vi "Write to File.vi"(8 "error in (no error)":errorcluster, 10 "INI Ref":T1, 11 "Window Action in":refnum<class "Window Action.lvclass">) -> (0 "error out":errorcluster, 2 "INI Ref out":T1, 3 "Window Action out":refnum<class "Window Action.lvclass">)   [LabVIEW 2020, in "MacroAssert.lvlib" / "Window Action.lvclass"]
doc: "Writes associated parameters to the file identified by <B>INI Ref</B>."
uses:
  Window Action.lvclass
  C:/Users/User/Documents/LabVIEW Data/Projects/MacroAssert/source/Classes/Step/Step.lvclass
  <vilib>/Utility/config.llb/Config Data RefNum.ctl
  <vilib>/Utility/error.llb/Error Cluster From Error Code.vi
  <vilib>/Utility/config.llb/Write Key (String).vi
  Action Step/Action Step.lvclass
  MacroAssert.lvlib
  <vilib>/Utility/config.llb/NI_LVConfig.lvlib
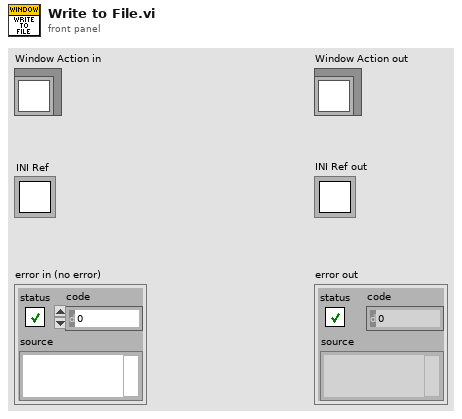
[diagram p1: front panel]
types:
  T1 = typedef "NI_LVConfig.lvlib/Config Data RefNum.ctl" = refnum<k1>
  T2 = typedef "MacroAssert.lvlib/Window Action.lvclass/Window Action Type.ctl" = enum16{"Maximize Window", "Restore Window", "Minimize Window", "Close Window", "Bring Window to Front", "Send Window to Back"}
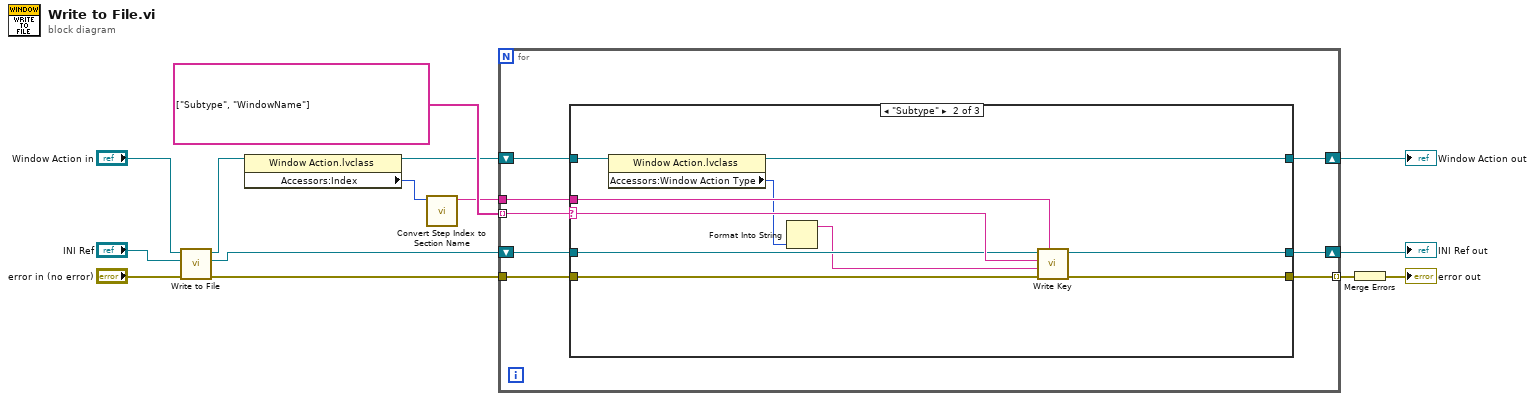
[diagram p0: block diagram]
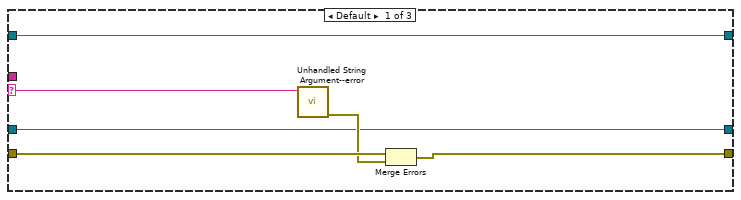
[diagram p2: hidden frame]
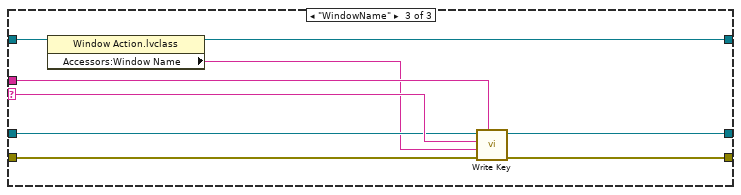
[diagram p3: hidden frame]
diagram:
  n1 = call-parent "Write to File.vi"("error in (no error)"="error in (no error)", "INI Ref"="INI Ref", "Step in"="Window Action in") -> ("error out"=w9:errorcluster, "INI Ref out"=w7:T1, "Step out"=w8:refnum<class "Window Action.lvclass">)  [unwired: 6 in]
  n2 = property class="Window Action.lvclass"(reference=w8) -> (reference out=w11:refnum<class "Window Action.lvclass">, "Accessors:Index"=w14:i32)  [unwired: 1 in, 1 out]
  n3 = call "Convert Step Index to Section Name.vi"("Step Index"=w14) -> ("Section Name"=w10:string)  [unwired: 10 in]
  n4 = for {
    tunnel: string[] ["Subtype", "WindowName"] -> [w22] mode=indexing
    tunnel: w9 -> [w21]
    tunnel: w10 -> [w20]
    shift-right: [w18] -> w3
    shift-left: w11 -> [w19]
    tunnel: [w17] -> w12 mode=indexing
    shift-right: [w15] -> w1
    shift-left: w7 -> [w16]
    n5 = case shown="\"Subtype\"" w22 {
      selector: w22 -> [w25 w36 w45]
      tunnel: w21 -> [w27 w38 w47]
      tunnel: w20 -> [_ w37 w46]
      tunnel: w19 -> [w28 w34 w43]
      tunnel: [w28 w29 w40] -> w18
      tunnel: [w24 w33 w42] -> w17
      tunnel: w16 -> [w23 w35 w44]
      tunnel: [w23 w32 w41] -> w15
      frame Default {
        n6 = call "Unhandled String Argument--error.vi"("Argument"=w25) -> ("error out"=w26:errorcluster)  [unwired: 10 in]
        n7 = Merge Errors(w27, w26) -> (w24:errorcluster)
      }
      frame "Subtype" {
        n8 = property class="Window Action.lvclass"(reference=w34) -> (reference out=w29:refnum<class "Window Action.lvclass">, "Accessors:Window Action Type"=w31:T2)  [unwired: 1 in, 1 out]
        n9 = Format Into String(w31) -> (resulting string=w30:string)  [unwired: 3 in, 1 out]
        n10 = call-poly <vilib>:"Write Key.vi"("section"=w37, "error in (no error)"=w38, "value"=w30, "key"=w36, "refnum"=w35) -> ("error out"=w33:errorcluster, "refnum out"=w32:T1)  [unwired: 4 in, 1 out]
      }
      frame "WindowName" {
        n11 = property class="Window Action.lvclass"(reference=w43) -> (reference out=w40:refnum<class "Window Action.lvclass">, "Accessors:Window Name"=w39:string)  [unwired: 1 in, 1 out]
        n12 = call-poly <vilib>:"Write Key.vi"("section"=w46, "error in (no error)"=w47, "value"=w39, "key"=w45, "refnum"=w44) -> ("error out"=w42:errorcluster, "refnum out"=w41:T1)  [unwired: 4 in, 1 out]
      }
    }
  }
  "Window Action out" <- w3
  "INI Ref out" <- w1
  n13 = Merge Errors(w12) -> (→"error out":errorcluster)
